vi "Convert Controls to Cluster.vi"(11 "Control Array":string[][](array[string])) -> (3 "Ctl Properties":T1[](array[typedef]))   [LabVIEW 2023, in "VI Properties Editor.lvlib"]
doc: "Converts <B>Control Array</B> and <B>Indicator Array</B> to a cluster array to be used by back-end processes."
uses:
  VI Properties Editor.lvlib
  CTLs/Control Properties.ctl
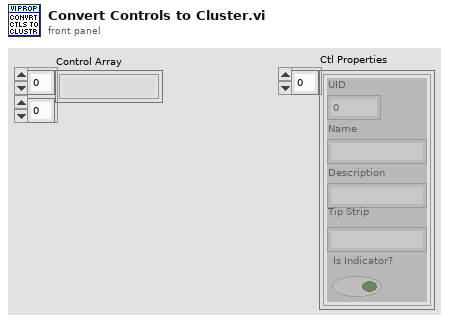
[diagram p1: front panel]
types:
  T1 = typedef "VI Properties Editor.lvlib/Control Properties.ctl" = cluster{"UID":i32, "Name":string, "Description":string, "Tip Strip":string, "Is Indicator?":bool}
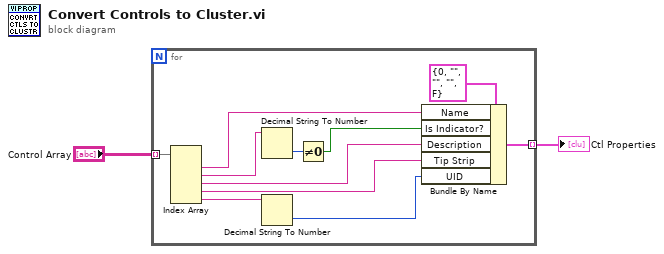
[diagram p0: block diagram]
diagram:
  n1 = for {
    tunnel: "Control Array" -> [w12] mode=indexing
    tunnel: [w10] -> w1 mode=indexing
    n2 = Index Array(array=w12) -> (element #1=w11:string, element #2=w9:string, element #3=w6:string, element #4=w5:string, element #5=w4:string)  [unwired: 5 in]
    n3 = Decimal String To Number(string=w9) -> (number=w8:i32)  [unwired: 2 in, 1 out]
    n4 = Decimal String To Number(string=w4) -> (number=w3:i32)  [unwired: 2 in, 1 out]
    n5 = Not Equal To 0?(x=w8) -> (x != 0?=w7:bool)
    n6 = Bundle By Name(cluster=T1 {"UID"=0, "Name"="", "Description"="", "Tip Strip"="", "Is Indicator?"=FALSE} ("input cluster"), "Name"=w11, "Is Indicator?"=w7, "Description"=w6, "Tip Strip"=w5, "UID"=w3) -> (w10:T1)
  }
  "Ctl Properties" <- w1
